vi "UART.vi"() -> ()   [LabVIEW 2019]
uses:
  <vilib>/myRIO/Instrument Drivers/Onboard IO/UART/typedef/VISA Configuration.ctl
  <vilib>/Utility/error.llb/Error Cluster From Error Code.vi
  <vilib>/myRIO/Common/Instrument Driver Framework/ELVIS III v1.0/ELVIS III v1.1 Open.vi
  <vilib>/myRIO/Common/Instrument Driver Framework/ELVIS III v1.0/Resource Manager/vis/ELVIS III v1.0 Reserve Channel List.vi
  <vilib>/myRIO/Common/Instrument Driver Framework/myRIO v1.0/myRIO v1.0 Close.vi
  <vilib>/Instr/_visa.llb/VISA Configure Serial Port (Instr).vi
  <vilib>/myRIO/Common/Instrument Driver Framework/Utilities/vis/FPGA Ref Manager.vi
  <vilib>/myRIO/Common/Instrument Driver Framework/ELVIS III v1.0/Resource Manager/vis/ELVIS III v1.0 Unreserve Channel List.vi
  <vilib>/myRIO/Common/Instrument Driver Framework/ELVIS III v1.0/ELVIS III v1.0 Reset FPGA.vi
  <vilib>/myRIO/Common/Instrument Driver Framework/myRIO v1.0/IRQ/vis/myRIO v1.0 IRQ Info FGV.vi
  <vilib>/myRIO/Common/Instrument Driver Framework/myRIO v1.0/IRQ/vis/myRIO v1.0 Timer IRQ Info FGV.vi
  <vilib>/myRIO/Common/Instrument Driver Framework/myRIO v1.0/IRQ/vis/myRIO v1.0 ISR Agent.vi
  <vilib>/myRIO/Instrument Drivers/Utilities/vis/Reset Index.vi
  <vilib>/myRIO/Common/Instrument Driver Framework/myRIO v1.0/Resource Manager/vis/myRIO v1.0 Block Write Resource Manager.vi
  <vilib>/myRIO/Instrument Drivers/Utilities/Utilities.lvlib
  <vilib>/myRIO/Instrument Drivers/Onboard IO/UART/UART.lvlib
panel:
  out "Characters Read":string
  out "Character Count":u32
  in  "Characters to Write":string="Example string."
  # "ELVIS III Control IO"
  # "UART"
  # "Overview: Performs a loopback test on the Bank A UART lines (RX: A/DIO16, TX: A/DIO17).\nInstructions:\n1. Connect a wire from A/DIO16 to A/DIO17.\n2. Change the text within the Characters to Write.\n3. Run the VI.\n4. Notice Characters Read contains the same characters written to Characters to Write."
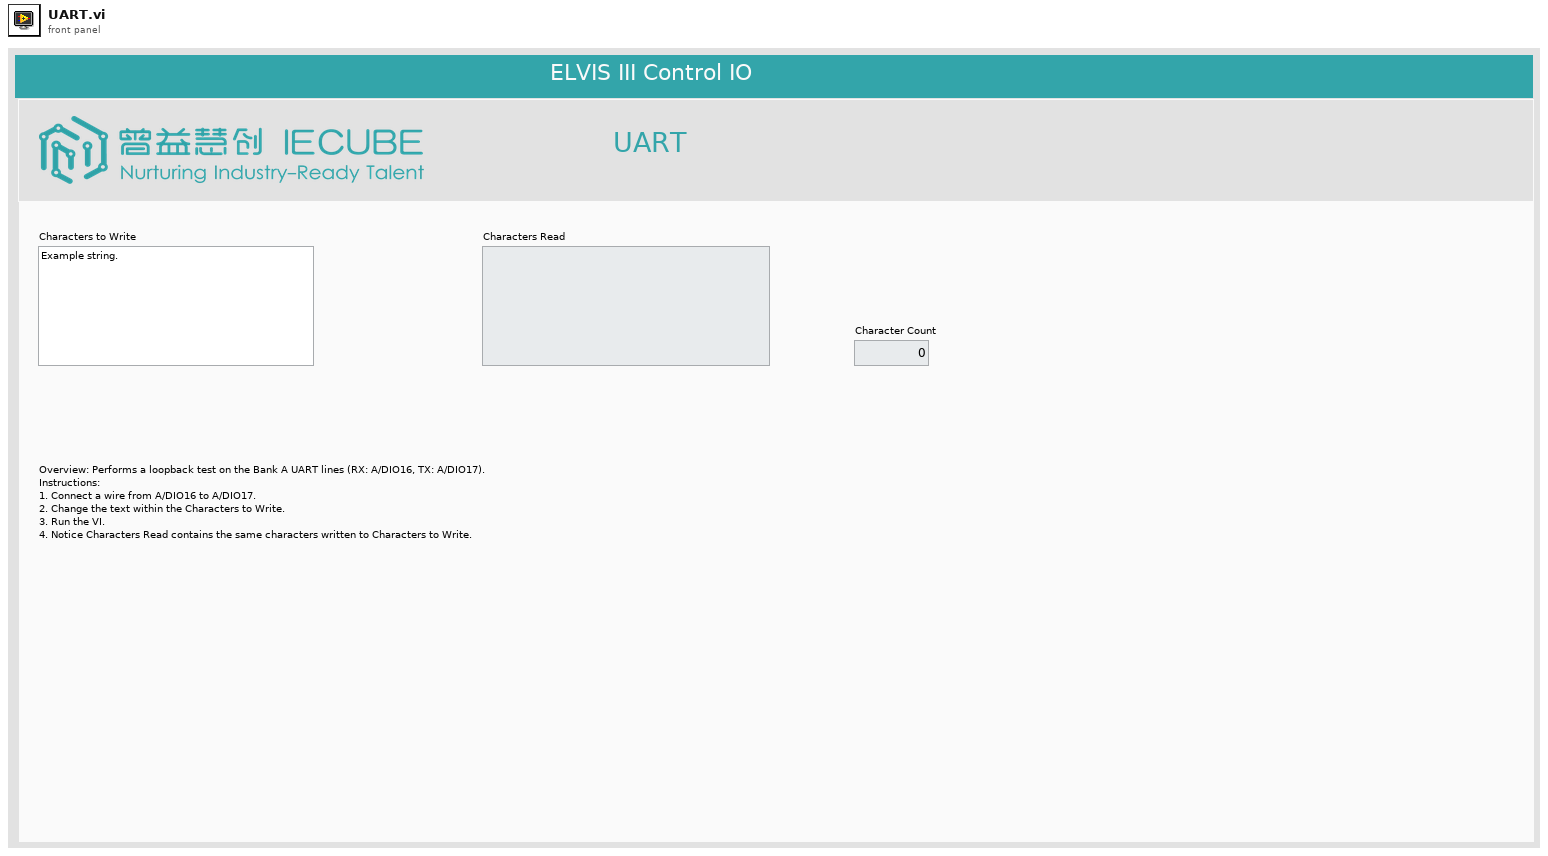
[diagram p1: front panel]
types:
  T1 = typedef "UART.lvlib/VISA Configuration.ctl" = cluster{"baud rate (9600)":u32, "data bits (8)":u16, "parity (0:none)":enum16{"None", "Odd", "Even", "Mark", "Space"}, "stop bits (10: 1 bit)":u16, "flow control (0:none)":u16, "termination char\n(0xA = '\\n' = LF) ":u8, "Enable Termination\nChar (T)":bool, "timeout (10sec)":u32}
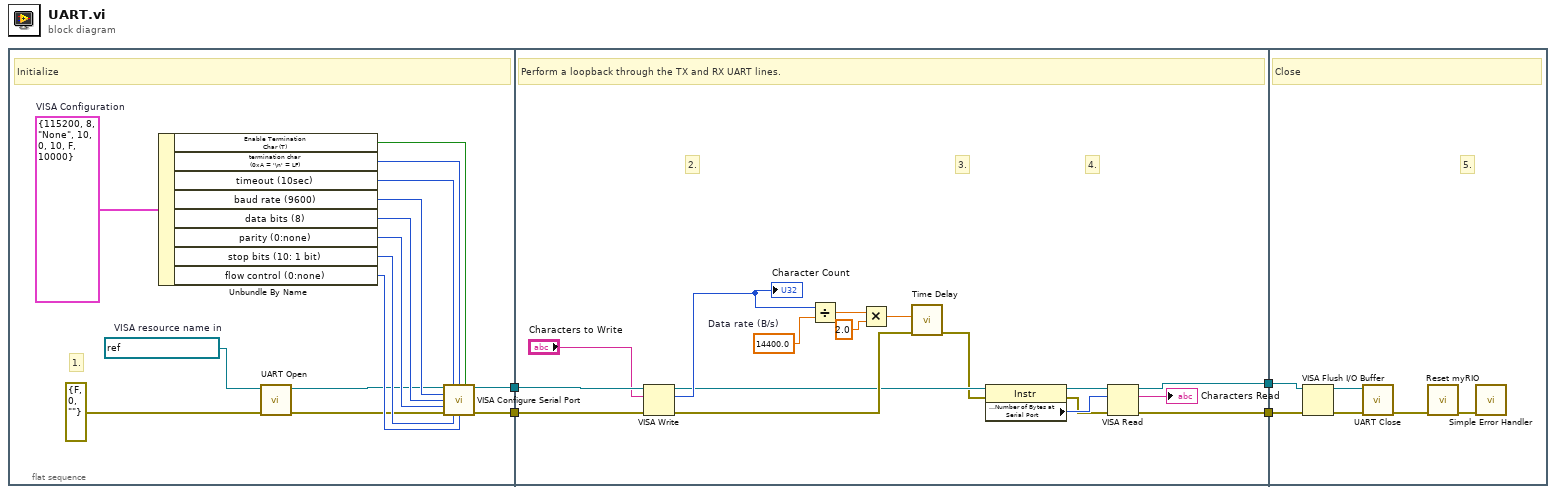
[diagram p0: block diagram]
diagram:
  n1 = flat-sequence {
    tunnel: [w6] -> w3
    tunnel: [w5] -> w2
    tunnel: [w21] -> w4
    tunnel: w3 -> [w32]
    tunnel: w2 -> [w31]
    tunnel: [w20] -> w1
    tunnel: w4 -> [w39]
    tunnel: w1 -> [w37]
    frame #0 {
      w9 = T1 {"baud rate (9600)"=115200, "data bits (8)"=8, "parity (0:none)"=enum."None", "stop bits (10: 1 bit)"=10, "flow control (0:none)"=0, "termination char\n(0xA = '\\n' = LF) "=10, "Enable Termination\nChar (T)"=FALSE, "timeout (10sec)"=10000}  # VISA Configuration
      w8 = refnum<visa-resource-name> "ASRL1::INSTR"  # VISA resource name in
      # "1."
      # "Initialize"
      n2 = Unbundle By Name(w9) -> ("Enable Termination\nChar (T)"=w12:bool, "termination char\n(0xA = '\\n' = LF)"=w13:u8, "timeout (10sec)"=w14:u32, "baud rate (9600)"=w19:u32, "data bits (8)"=w18:u16, "parity (0:none)"=w17:enum16{"None", "Odd", "Even", "Mark", "Space"}, "stop bits (10: 1 bit)"=w16:u16, "flow control (0:none)"=w15:u16)
      n3 = call <vilib>:"UART Open.vi"("error in (no error)"=errorcluster {"status"=FALSE, "code"=0, "source"=""} ("Error In"), "VISA resource name in"=w8) -> ("error out"=w11:errorcluster, "VISA resource name out"=w10:refnum<visa-resource-name>)  [unwired: 8 in]
      n4 = call-poly "VISA Configure Serial Port"("VISA resource name"=w10, "timeout (10sec)"=w14, "termination char\n(0xA = '\\n' = LF)"=w13, "Enable Termination\nChar (T)"=w12, "baud rate (9600)"=w19, "data bits (8)"=w18, "parity (0:none)"=w17, "error in (no error)"=w11, "stop bits (10: 1 bit)"=w16, "flow control (0:none)"=w15) -> ("VISA resource name out"=w5:refnum<visa-resource-name>, "error out"=w6:errorcluster)  [unwired: 4 in]
    }
    frame #1 {
      w35 = 14400.0  # Data rate (B/s)
      # "4."
      # "3."
      # "2."
      # "Perform a loopback through the TX and RX UART lines."
      n5 = VISA Write(VISA resource name=w31, write buffer="Characters to Write", error in (no error)=w32) -> (VISA resource name out=w25:refnum<visa-resource-name>, return count=w29:u32, error out=w28:errorcluster)
      "Character Count" <- w29
      n6 = Divide(x=w29, y=w35) -> (x/y=w36:dbl)
      n7 = Multiply(x=w36, y=2.0) -> (x*y=w33:dbl)
      n8 = call "Time Delay"("error in (no error)"=w28, "Delay Time (s)"=w33) -> ("error out"=w23:errorcluster)  [unwired: 9 in]
      n9 = property class="Instr"(reference=w25, error in=w23) -> (reference out=w27:refnum<visa-resource-name>, error out=w22:errorcluster, "Serial Settings:Number of Bytes at Serial Port"=w26:u32)
      n10 = VISA Read(VISA resource name=w27, byte count=w26, error in (no error)=w22) -> (VISA resource name out=w20:refnum<visa-resource-name>, read buffer=→"Characters Read":string, error out=w21:errorcluster)  [unwired: 1 out]
    }
    frame #2 {
      # "5."
      # "Close"
      n11 = VISA Flush I/O Buffer(VISA resource name=w37, error in (no error)=w39) -> (VISA resource name out=w41:refnum<visa-resource-name>, error out=w40:errorcluster)  [unwired: 1 in]
      n12 = call <vilib>:"UART Close.vi"("error in (no error)"=w40, "VISA resource name in"=w41) -> ("error out"=w38:errorcluster)  [unwired: 9 in]
      n13 = call <vilib>:"Reset myRIO.vi"("error in (no error)"=w38) -> ("error out"=w42:errorcluster)  [unwired: 10 in]
      n14 = call <vilib>:"Simple Error Handler.vi"("error in (no error)"=w42) -> ()  [unwired: 4 in, 5 out]
    }
  }
